vi "Read NI_API_ConnectionRef.vi"(8 "error in (no error)":errorcluster, 11 "NI_DB_API in":refnum<class "NI_DB_API.lvclass">) -> (0 "error out":errorcluster, 2 "reference":T1, 3 "NI_DB_API out":refnum<class "NI_DB_API.lvclass">)   [LabVIEW 2021, in "NI_DB_API.lvclass"]
uses:
  <userlib>/John_Lib/DataBase/NI_DB_API/NI_DB_API.lvclass
  <userlib>/John_Lib/DataBase/NI_DB_API/NI_DB_API.lvclass/NI_DB_API.ctl
  <vilib>/addons/database/Connection.llb/Conn ObjectReference.ctl
  <vilib>/addons/database/NI_Database_API.lvlib
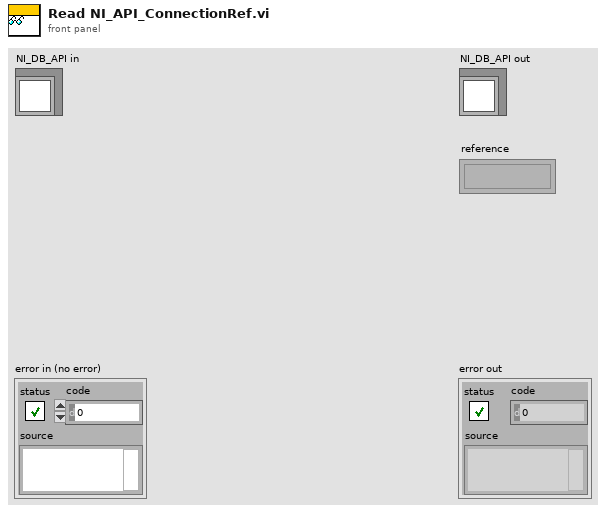
[diagram p1: front panel]
types:
  T1 = typedef "NI_Database_API.lvlib/Conn ObjectReference.ctl" = refnum<k1>
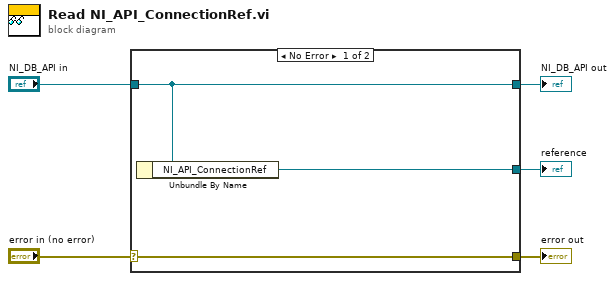
[diagram p0: block diagram]
diagram:
  n1 = case shown="No Error" "error in (no error)" {
    selector: "error in (no error)" -> [w8 w9]
    tunnel: [w8 w9] -> w4
    tunnel: [w7 w10] -> w2
    tunnel: "NI_DB_API in" -> [w7 w10]
    tunnel: [w6 _] -> w1
    frame No Error {
      n2 = Unbundle By Name(w7) -> ("NI_API_ConnectionRef"=w6:T1)
    }
    frame Error {
    }
  }
  "error out" <- w4
  "NI_DB_API out" <- w2
  "reference" <- w1
